vi "Measure Output.vi"(8 "error in":errorcluster, 11 "89XX in":refnum<class "89XX.lvclass">) -> (0 "error out":errorcluster, 1 "Current":dbl[](array[numeric]), 2 "Voltage":dbl[](array[numeric]), 3 "89XX out":refnum<class "89XX.lvclass">)   [LabVIEW 2019, in "89XX.lvlib" / "89XX.lvclass"]
doc: "Child classes must override this VI:\n\nThis VI is the device specific query of current and voltage measurements. \nThe return values are: \nVoltage Array - One voltage measurement per channel single channel supplies should only return a single array element\nCurrent Array - - One current measurement per channel single channel supplies should only return a single array element"
uses:
  Library/89XX.lvclass
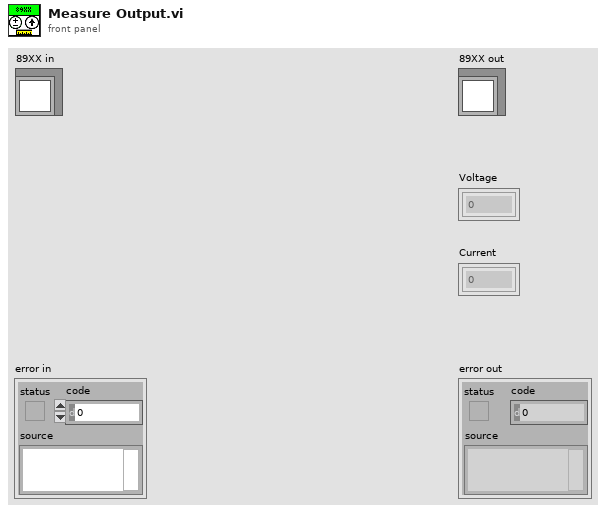
[diagram p1: front panel]
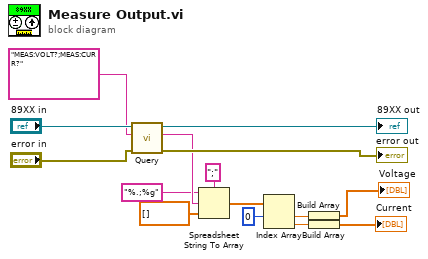
[diagram p0: block diagram]
diagram:
  n1 = call "Query.vi"("error in"="error in", "Query"="MEAS:VOLT?;MEAS:CURR?", "89XX in"="89XX in") -> ("error out"=→"error out":errorcluster, "Response"=w10:string, "89XX out"=→"89XX out":refnum<class "89XX.lvclass">)  [unwired: 6 in]
  n2 = Spreadsheet String To Array(delimiter (Tab)=";", format string="%.;%g", spreadsheet string=w10, array type (2D Dbl)=dbl[] []) -> (array=w6:dbl[])
  n3 = Index Array(array=w6, index #1=0 ("index")) -> (element #1=w3:dbl, element #2=w4:dbl)  [unwired: 1 in]
  n4 = Build Array(w3) -> (→"Voltage":dbl[])
  n5 = Build Array(w4) -> (→"Current":dbl[])
